vi "Read DI Array.vi"(8 "error in (no error)":errorcluster, 11 "FPGA in":refnum<class "FPGA.lvclass">) -> (0 "error out":errorcluster, 2 "DI array":bool[](array[boolean]), 3 "FPGA out":refnum<class "FPGA.lvclass">)   [LabVIEW 2019, in "FPGA.lvclass"]
uses:
  FPGA.lvclass
  FPGA.lvclass/FPGA.ctl
  <vilib>/Utility/error.llb/Error Cluster From Error Code.vi
  <vilib>/rvi/errors/niLvFpgaAdjustHostInterfaceError.vi
  <vilib>/rvi/interface/nirviReadWriteControl/nirviReadWriteControl.xnode
  FPGA VI Reference.ctl
  NiFpgaLv.dll
  <vilib>/rvi/interface/Simulation/niFpgaSimulationCallBeginRW.vi
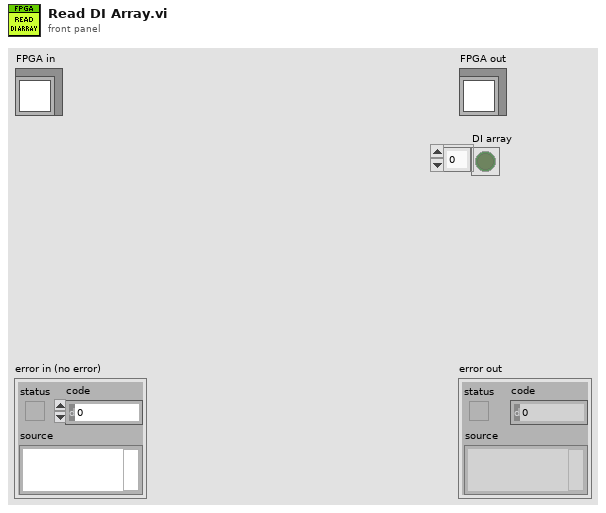
[diagram p1: front panel]
types:
  T1 = typedef "FPGA.lvclass/FPGA VI Reference.ctl" = refnum<k20>
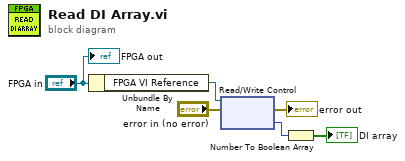
[diagram p0: block diagram]
diagram:
  n1 = Unbundle By Name("FPGA in") -> ("FPGA VI Reference"=w5:T1)
  n2 = xnode "Read/Write Control"("FPGA VI Reference In"=w5, "error in"="error in (no error)") -> ("error out"=→"error out":errorcluster, "DIs"=w3:u32)  [unwired: 1 out]
  n3 = Number To Boolean Array(number=w3) -> (Boolean array=→"DI array":bool[])
  "FPGA out" <- "FPGA in"
